vi "Write-Read Text File.vi"() -> ()   [LabVIEW 2009]
doc: "This example shows how the Write and Read Text File functions operate using different options. Click the Run button to execute and examine the behavior of each case."
uses:
  <vilib>/Instr/_visa.llb/VISA Configure Serial Port (Instr).vi
panel:
  in  "XON Character":u8=17 format="%.0x"
  in  "XOFF Character":u8=19 format="%.0x"
  in  "flow control":u16(ring) items=["None"=0, "XON/XOFF"=1, "RTS/CTS"=2, "DTR/DSR"=4]
  in  "End write with termination character?":bool=TRUE
  in  "Input\nbuffer size":u32=4096
  in  "stop":bool
  in  "termination char\n(0xA = '\\n' = LF)":u8=10 format="%.0x"
  in  "End read on termination character?":bool=TRUE
  in  "timeout (ms)":u32=10000
  in  "stop bits":u16(ring)=10 items=["1.0"=10, "1.5"=15, "2.0"=20]
  in  "parity":u16(ring) items=["None", "Odd", "Even", "Mark", "Space"]
  in  "data bits":u16=8 min=5 max=8 step=1
  in  "VISA resource name":refnum<visa-resource-name>="COM1"
  in  "baud rate":u32=115200
  out "Read Text 2":string
  in  "Path 2":path=path "C:/Users/LSI/Documents/MATLAB/XYplotter/matlab/EdgeData.txt"
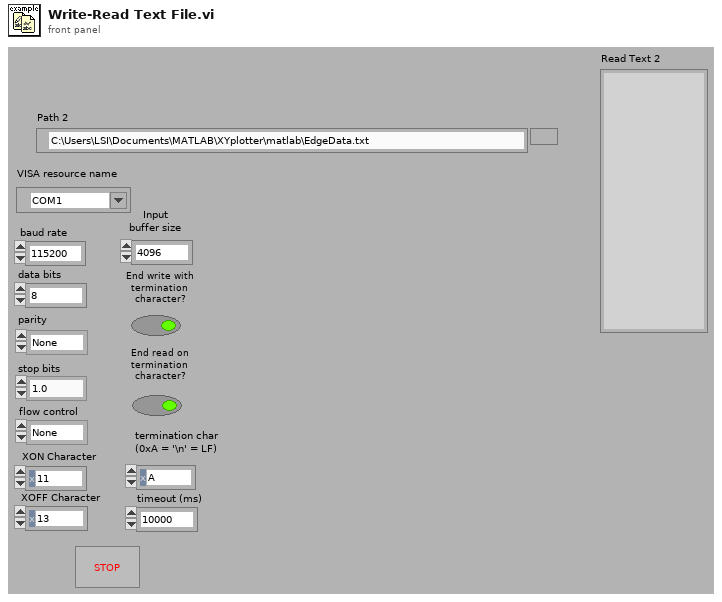
[diagram p1: front panel]
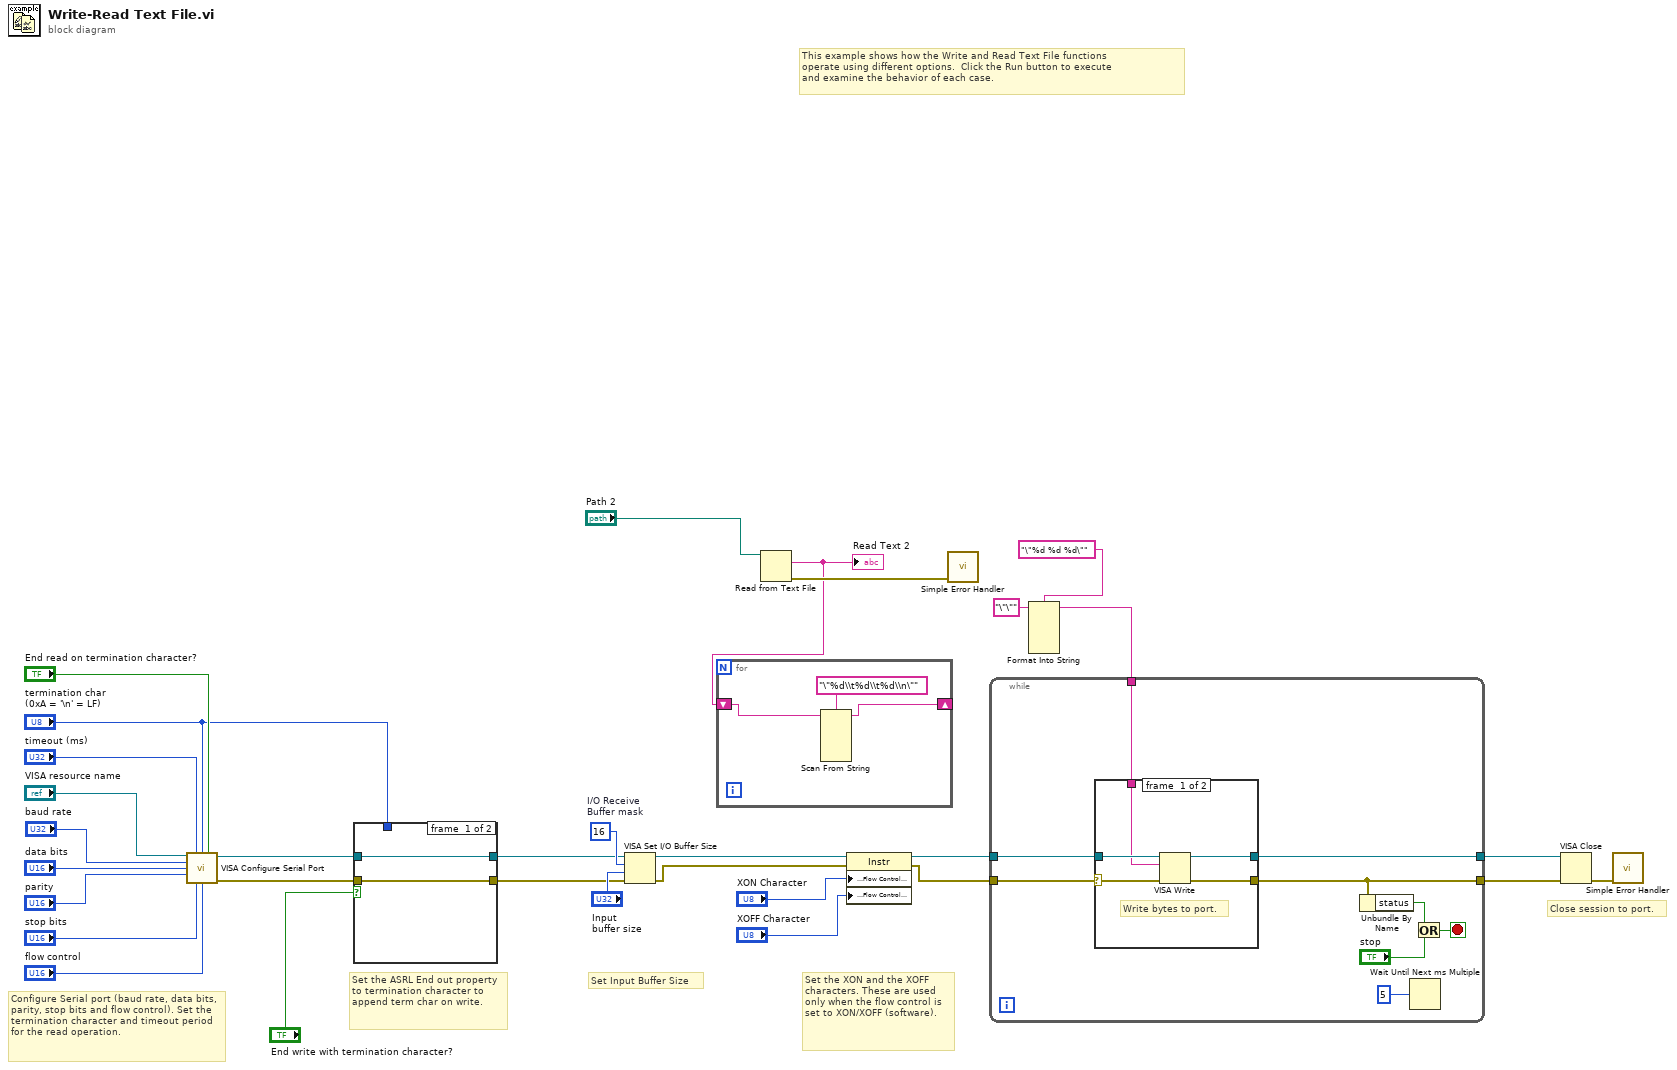
[diagram p0: block diagram]
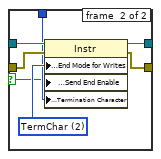
[diagram p2: hidden frame]
diagram:
  w22 = u16 16  # I/O Receive Buffer mask
  # "Set the XON and the XOFF characters. These are used only when the flow control is set to XON/XOFF (software)."
  # "Configure Serial port (baud rate, data bits, parity, stop bits and flow control). Set the termination character and timeout period for the read operation."
  # "Set Input Buffer Size"
  # "Set the ASRL End out property to termination character to append term char on write."
  # "Close session to port."
  # "This example shows how the Write and Read Text File functions \noperate using different options.  Click the Run button to execute \nand examine the behavior of each case."
  n1 = call-poly "VISA Configure Serial Port"("VISA resource name"="VISA resource name", "timeout (10sec)"="timeout (ms)", "termination char\n(0xA = '\\n' = LF)"="termination char\n(0xA = '\\n' = LF)", "Enable Termination\nChar (T)"="End read on termination character?", "baud rate (9600)"="baud rate", "data bits (8)"="data bits", "parity (0:none)"="parity", "stop bits (10: 1 bit)"="stop bits", "flow control (0:none)"="flow control") -> ("VISA resource name out"=w8:refnum<visa-resource-name>, "error out"=w11:errorcluster)  [unwired: 1 in, 4 out]
  n2 = case shown="True" "End write with termination character?" {
    selector: "End write with termination character?" -> [_ w34]
    tunnel: w8 -> [w32 w40]
    tunnel: w11 -> [w33 w39]
    tunnel: [w32 w38] -> w9
    tunnel: [w33 w37] -> w10
    tunnel: "termination char\n(0xA = '\\n' = LF)" -> [_ w35]
    frame #0 {
    }
    frame #1 {
      w36 = u16 2 items=["None", "LastBit", "TermChar", "Break"] ("Serial Settings:Serial End Mode for Writes")
      n3 = property class="Instr"(reference=w40, error in=w39, "Serial Settings:End Mode for Writes"=w36, "Message Based Settings:Send End Enable"=w34, "Message Based Settings:Termination Character"=w35) -> (reference out=w38:refnum<visa-resource-name>, error out=w37:errorcluster)
    }
  }
  n4 = VISA Set I/O Buffer Size(VISA resource name=w9, mask (16)=w22, size (4096)="Input\nbuffer size", error in (no error)=w10) -> (VISA resource name out=w17:refnum<visa-resource-name>, error out=w16:errorcluster)
  n5 = Read from Text File(file (use dialog)="Path 2") -> (text=w4:string, error out=w30:errorcluster)  [unwired: 3 in, 2 out]
  "Read Text 2" <- w4
  n6 = for {
    shift-right: [w41] -> _
    shift-left: w4 -> [w42]
    n7 = Scan From String(format string="\"%d\\t%d\\t%d\\n\"", input string=w42) -> (remaining string=w41:string)  [unwired: 8 in, 2 out]
  }
  n8 = property class="Instr"(reference=w17, error in=w16, "Serial Settings:Flow Control XON Character"="XON Character", "Serial Settings:Flow Control XOFF Character"="XOFF Character") -> (reference out=w7:refnum<visa-resource-name>, error out=w13:errorcluster)
  n9 = call <vilib>:"Simple Error Handler.vi"("error in (no error)"=w30) -> ()  [unwired: 4 in, 5 out]
  n10 = Format Into String(format string="\"%d %d %d\"", initial string="\"\"") -> (resulting string=w3:string)  [unwired: 5 in, 1 out]
  n11 = while {
    tunnel: w13 -> [w45]
    tunnel: w7 -> [w46]
    tunnel: [w48] -> w6
    tunnel: [w47] -> w5
    tunnel: w3 -> [w44]
    stop <- w50 stop-if-true
    n12 = case shown="No Error" w45 {
      selector: w45 -> [w54 w59]
      tunnel: [w57 w58] -> w48
      tunnel: [w56 w59] -> w47
      tunnel: w46 -> [w55 w58]
      tunnel: w44 -> [w53 _]
      frame #0 {
        # "Write bytes to port."
        n13 = VISA Write(VISA resource name=w55, write buffer=w53, error in (no error)=w54) -> (VISA resource name out=w57:refnum<visa-resource-name>, error out=w56:errorcluster)  [unwired: 1 out]
      }
      frame #1 {
      }
    }
    n14 = Unbundle By Name(w47) -> ("status"=w51:bool)
    n15 = Wait Until Next ms Multiple(millisecond multiple=u32 5) -> ()  [unwired: 1 out]
    n16 = Or(x=w51, y="stop") -> (x .or. y?=w50:bool)
  }
  n17 = VISA Close(VISA resource name=w6, error in (no error)=w5) -> (error out=w27:errorcluster)
  n18 = call <vilib>:"Simple Error Handler.vi"("error in (no error)"=w27) -> ()  [unwired: 1 in, 8 out]
